vi "setLabel.vi"(6 "\"At\" location":T1, 7 "Justify":string(combo), 8 "Set?":bool=TRUE, 9 "multilineLabel":string[](array[string]), 10 "singleLabel":string, 11 "String in":string) -> (2 "command":string, 3 "String out":string)   [LabVIEW 2018]
uses:
  at.ctl
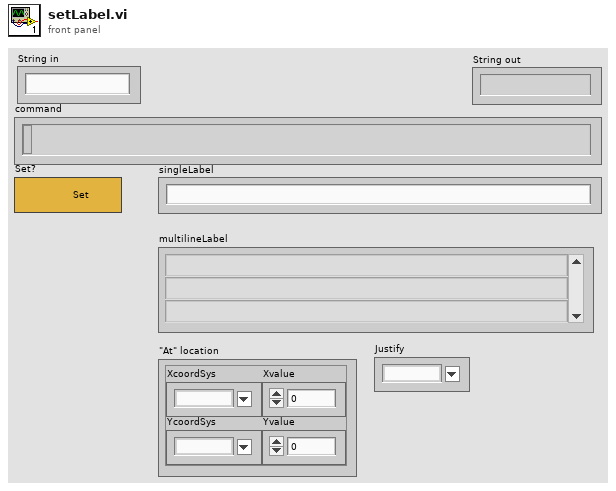
[diagram p1: front panel]
types:
  T1 = typedef "at.ctl" = cluster{"XcoordSys":string, "YcoordSys":string, "Xvalue":dbl, "Yvalue":dbl}
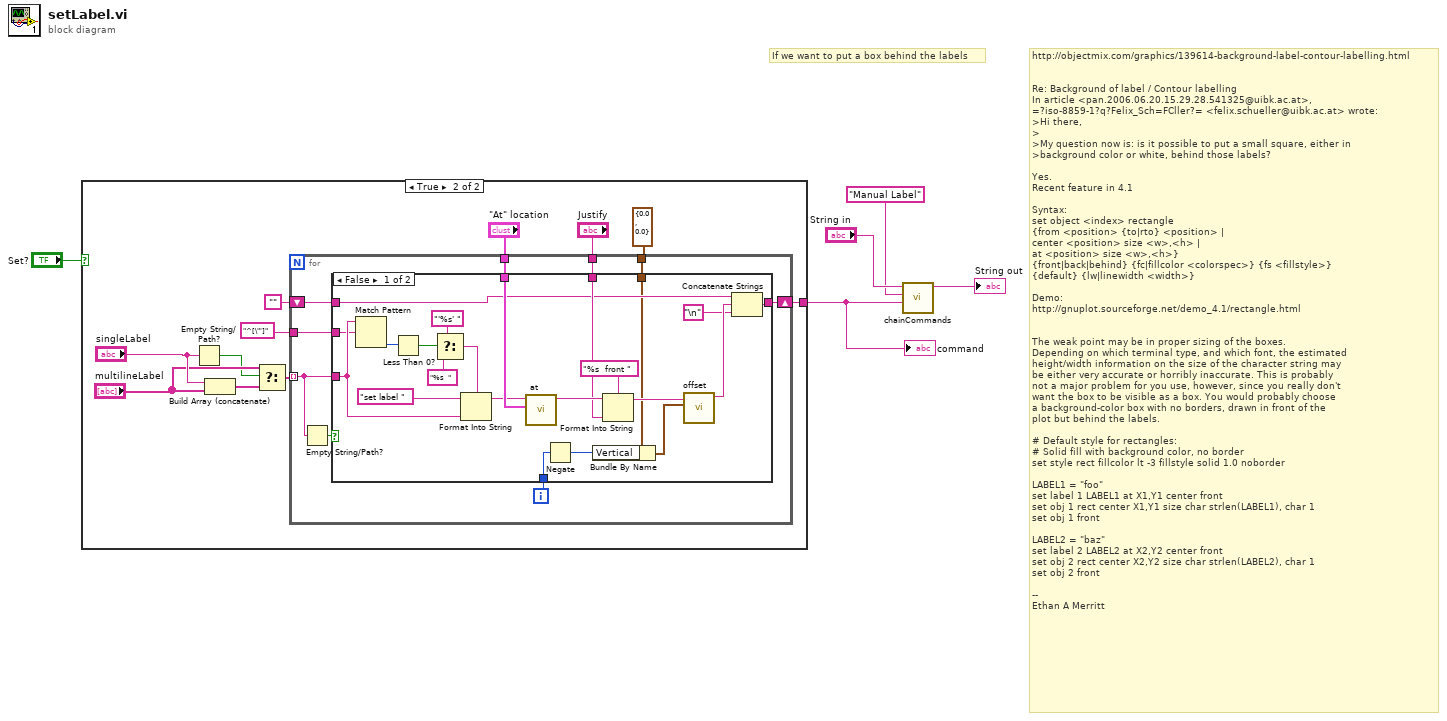
[diagram p0: block diagram]
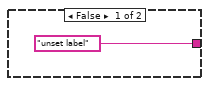
[diagram p2: hidden frame]
diagram:
  # "If we want to put a box behind the labels"
  # "http://objectmix.com/graphics/139614-background-label-contour-labelling.html\n\n\nRe: Background of label / Contour labelling\nIn article <pan.2006.06.20.15.29.28.541325@uibk.ac.at>,\n=?iso-8859-1?q?Felix_Sch=FCller?= <felix.schueller@uibk.ac.at> wrote:\n>Hi there,\n>\n>My question now is: is it possible to put a small square, either in\n>background color or white, behind those labels?\n\nYes.\nRecent feature in 4.1\n\nSyntax:\nset object <index> rectangle\n{from <position> {to|rto} <position> |\ncenter <position> size <w>,<h> |\nat <position> size <w>,<h>}\n{front|back|behind} {fc|fillcolor <colorspec>} {fs <fillstyle>}\n{default} {lw|linewidth <width>}\n\nDemo:\nhttp://gnuplot.sourceforge.net/demo_4.1/rectangle.html\n\n\nThe weak point may be in proper sizing of the boxes.\nDepending on which terminal type, and which font, the estimated\nheight/width information on the size of the character string may\nbe either very accurate or horribly inaccurate. This is probably\nnot a major problem for you use, however, since you really don't\nwant the box to be visible as a box. You would probably choose\na background-color box with no borders, drawn in front of the\nplot but behind the labels.\n\n# Default style for rectangles:\n# Solid fill with background color, no border\nset style rect fillcolor lt -3 fillstyle solid 1.0 noborder\n\nLABEL1 = \"foo\"\nset label 1 LABEL1 at X1,Y1 center front\nset obj 1 rect center X1,Y1 size char strlen(LABEL1), char 1\nset obj 1 front\n\nLABEL2 = \"baz\"\nset label 2 LABEL2 at X2,Y2 center front\nset obj 2 rect center X2,Y2 size char strlen(LABEL2), char 1\nset obj 2 front\n\n--\nEthan A Merritt"
  n1 = case shown="True" "Set?" {
    tunnel: ["unset label" w15] -> w3
    frame False {
    }
    frame True {
      n2 = Empty String/Path?(string/path="singleLabel") -> (empty?=w8:bool)
      n3 = Build Array (concatenate)("singleLabel", "multilineLabel") -> (w10:string[])
      n4 = Select(t="multilineLabel", s=w8, f=w10) -> (s? t:f=w12:string[])
      n5 = for {
        tunnel: "\"At\" location" -> [w26]
        tunnel: "Justify" -> [w25]
        shift-right: [w24] -> w15
        shift-left: "" -> [w23]
        tunnel: w12 -> [w19] mode=indexing
        tunnel: cluster{"Horizontal":dbl, "Vertical":dbl} {"Horizontal"=0.0, "Vertical"=0.0} ("offsetChars") -> [w21]
        tunnel: "^[\"']" ("regular expression") -> [w22]
        i -> [w20]
        n6 = Empty String/Path?(string/path=w19) -> (empty?=w18:bool)
        n7 = case shown="False" w18 {
          tunnel: w26 -> [w48 _]
          tunnel: w25 -> [w44 _]
          tunnel: [w36 w49] -> w24
          tunnel: w23 -> [w34 w49]
          tunnel: w19 -> [w33 _]
          tunnel: w22 -> [w31 _]
          tunnel: w21 -> [w30 _]
          tunnel: w20 -> [w29 _]
          frame False {
            n8 = Match Pattern(string=w33, regular expression=w31) -> (offset past match=w43:i32)  [unwired: 1 in, 3 out]
            n9 = Less Than 0?(x=w43) -> (x < 0?=w42:bool)
            n10 = Select(t="'%s' " ("format string"), s=w42, f="%s  " ("format string")) -> (s? t:f=w40:string)
            n11 = Format Into String(format string=w40, initial string="set label ", w33) -> (resulting string=w47:string)  [unwired: 1 in, 1 out]
            n12 = call "at.vi"("\"At\" location"=w48, "String in"=w47) -> ("String out"=w46:string)  [unwired: 9 in]
            n13 = Negate(x=w29) -> (-x=w27:i32)
            n14 = Bundle By Name(cluster=w30, "Vertical"=w27) -> (w28:cluster{"Horizontal":dbl, "Vertical":dbl})
            n15 = Format Into String(format string="%s  front ", initial string=w46, w44) -> (resulting string=w38:string)  [unwired: 1 in, 1 out]
            n16 = call "offset.vi"("offsetChars"=w28, "String in"=w38) -> ("String out"=w37:string)  [unwired: 9 in]
            n17 = Concatenate Strings(w34, w37, "\n" ("string")) -> (w36:string)
          }
          frame True {
          }
        }
      }
    }
  }
  "command" <- w3
  n18 = call "chainCommands.vi"("Command"=w3, "Comments"="Manual Label", "StringIn"="String in") -> ("StringOut"=→"String out":string)  [unwired: 8 in]
